vi "Synchronized Acquisition.vi"() -> ()   [LabVIEW 2021]
uses:
  <vilib>/userdefined/Silver/nirio_resource_slv.ctl
  Digitizer Control Class/Public/Acq Start Trigger Type.ctl
  <instrlib>/FlexRIO/API/Host/v1/NI FlexRIO/API/Reference Clock Source.ctl
  Digitizer Control Class/Public/TClk API Control Enable.ctl
  <instrlib>/FlexRIO/API/Host/v1/NI FlexRIO/API/Configure Reference Clock.vi
  <instrlib>/FlexRIO/API/Host/v1/NI FlexRIO API v1.lvlib
  <resource>/objmgr/sessionReference.rc
  Digitizer Control Class/Digitizer Control.lvclass
panel:
  out "Device Memory Utilization":u64[][](graph)
  out "Record index":i32
  in  "Acq # of records":i32=1
  out "actual pre-trigger period (s)":dbl format="%#_6p"
  in  "pre-trigger period (s)":dbl format="%#_6p"
  in  "Acq # of samples (per channel)":i64[](array[numeric])=[100000, 100000]
  in  "Enable Bit Packing (per channel)":bool[](array[boolean])=[FALSE, FALSE]
  in  "digital high level?":bool=TRUE
  in  "trigger type":T1
  in  "analog trigger channel":string="AI0"
  in  "analog/digital rising edge?":bool=TRUE
  in  "analog level (V)":dbl format="%#_3p"
  in  "analog hysteresis (V)":dbl format="%#_3p"
  in  "digital trigger source":string(combo)="DIO"
  out "Acq Overflow":bool[](array[boolean])
  in  "min. TClk period":dbl=1e-06 format="%#_6p"
  in  "trigger master index":i32
  out "Error Out":errorcluster
  in  "reference clock source":T2 items=["Default", "Onboard", "PXI_Clk10", "External", "None", "Baseboard Reference"]
  in  "Desired Sampling Rate (per device)":dbl[](array[numeric])=[800000000.0] format="%#_6p"
  out "Actual Sampling Rate (per device)":dbl[](array[numeric]) format="%#_6p"
  in  "AI channel":string="AI0,AI1"
  in  "devices":T3[](array[typedef])=["RIO0", "RIO1"]
  out "Power Spectrum":cluster{"f0":dbl, "df":dbl, "magnitude":dbl[]}[](graph) caption="Waveform Graph"
  in  "stop":bool
  out "Waveform Graph":waveform(dbl)[](graph)
  in  "TClk trigger\ncompensation?":bool
  # "Overview: Configure multiple 5774s for synchronized acquisition.\nRequirements: PXIe-5774 (KU060)\nInstructions: \n 1. Fill in the devices array with the resource name of the FlexRIO digitizers to synchronize.\n 2. Specify which device should be used as the trigger master using trigger master index\n 3. Configure the trigger settings for the master device\n 4. Optionally configure the reference clock to be used\n 5. Configure the channel to use, the number of samples and the sampling rate\n 5. Run the VI"
  # "Acquisition Trigger"
  # "Clocking configuration"
  # "Acquisition Configuration"
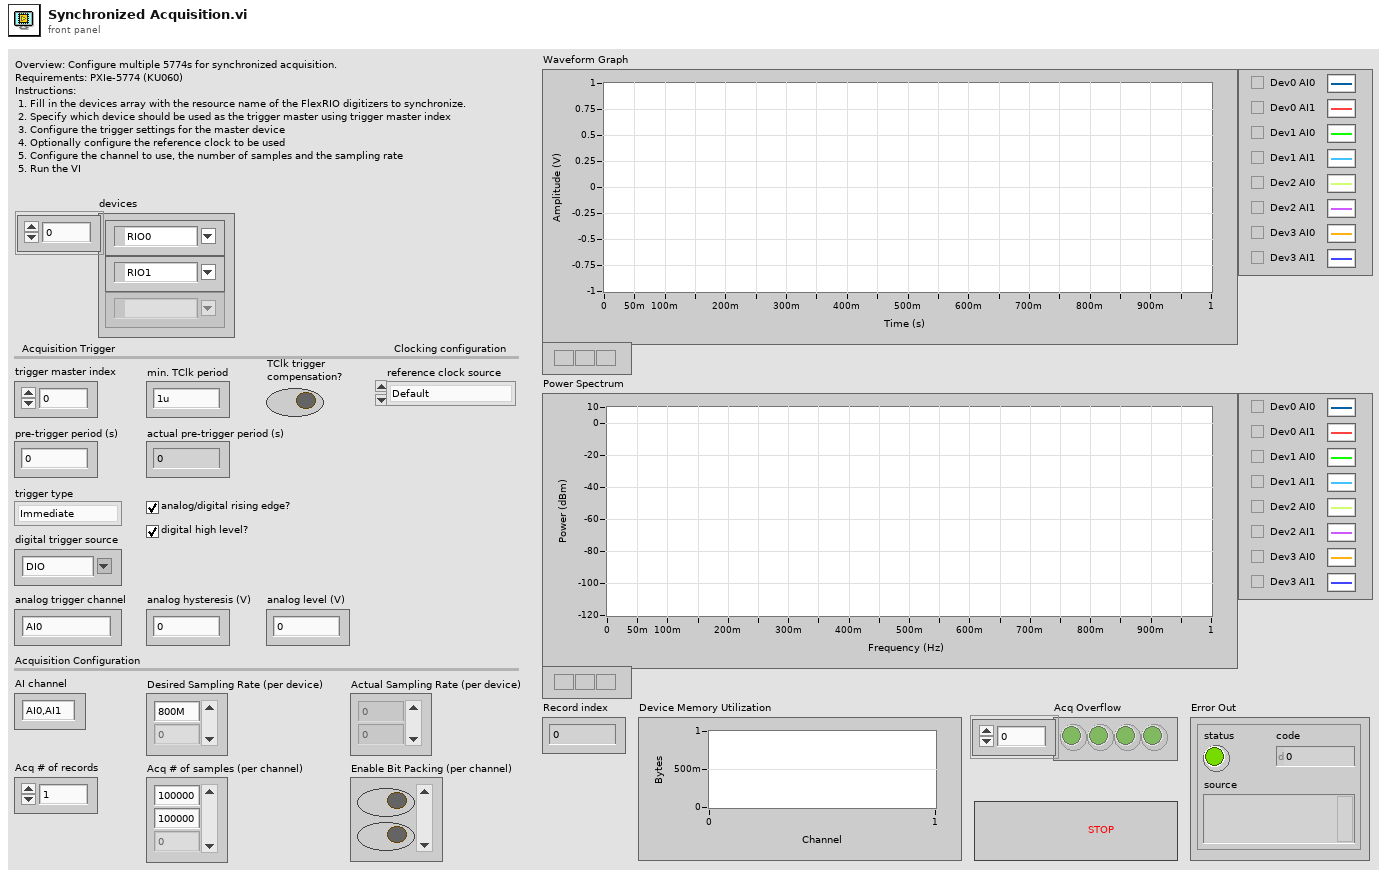
[diagram p1: front panel]
types:
  T1 = typedef "Digitizer Control.lvclass/Acq Start Trigger Type.ctl" = enum16{"Immediate", "Analog", "Digital Edge", "Digital Level"}
  T2 = typedef "NI FlexRIO API v1.lvlib/Reference Clock Source.ctl" = i32
  T3 = typedef "nirio_resource_slv.ctl" = tag
  T4 = typedef "Digitizer Control.lvclass/TClk API Control Enable.ctl" = enum16{"None", "Acquisition"}
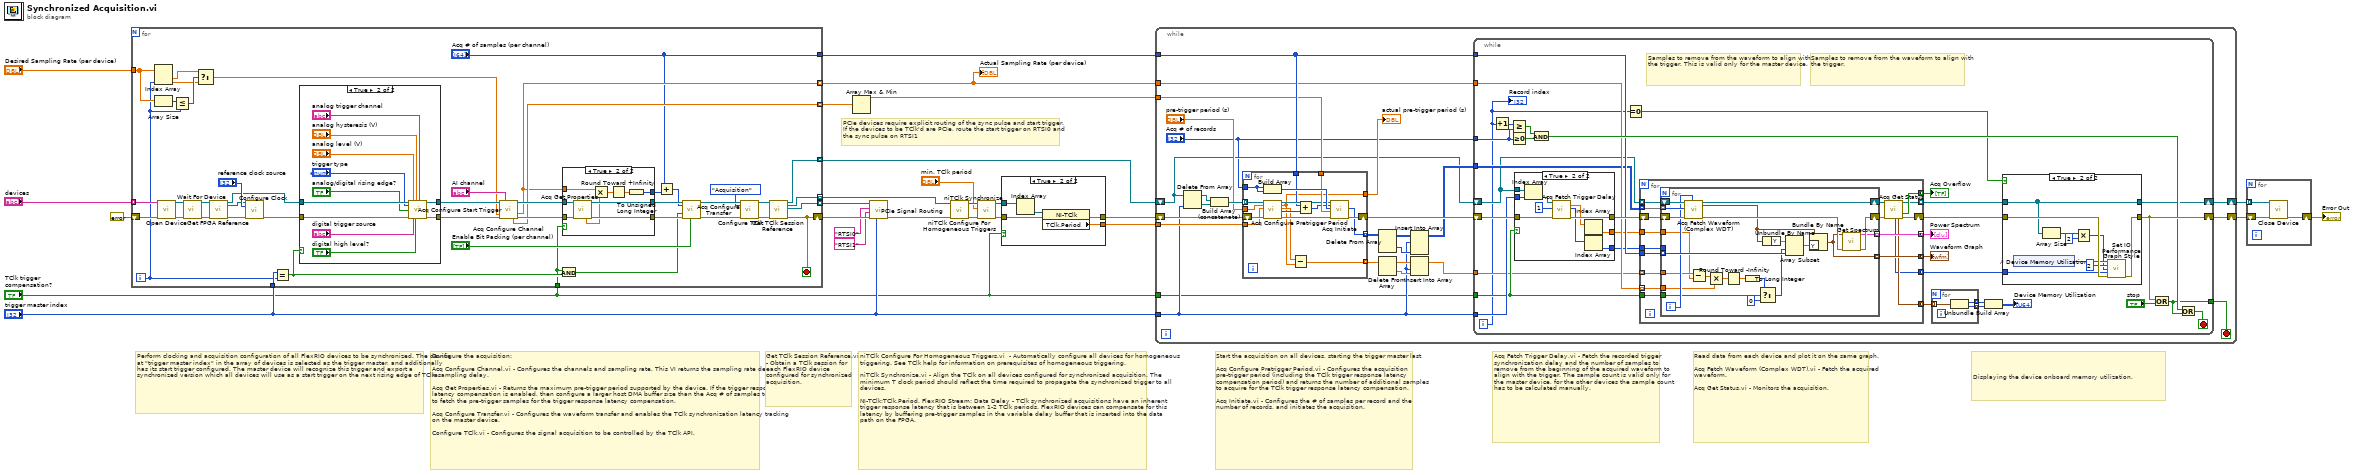
[diagram p0: block diagram]
diagram:
  # "Displaying the device onboard memory utilization."
  # "Read data from each device and plot it on the same graph.\n\nAcq Fetch Waveform (Complex WDT).vi - Fetch the acquired waveform.\n\nAcq Get Status.vi - Monitors the acquisition."
  # "Acq Fetch Trigger Delay.vi - Fetch the recorded trigger synchronization delay and the number of samples to remove from the beginning of the acquired waveform to align with the trigger. The sample count is valid only for the master device, for the other devices the sample count has to be calculated manually."
  # "Start the acquisition on all devices, starting the trigger master last\n\nAcq Configure Pretrigger Period.vi - Configures the acquisition pre-trigger period (including the TClk trigger response latency compensation period) and returns the number of additional samples to acquire for the TClk trigger response latency compensation.\n\nAcq Initiate.vi - Configures the # of samples per record and the number of records, and initiates the acquisition."
  # "Configure the acquisition:\n\nAcq Configure Channel.vi - Configures the channels and sampling rate. This VI returns the sampling rate dependent resampling delay.\n\nAcq Get Properties.vi - Returns the maximum pre-trigger period supported by the device. If the trigger response latency compensation is enabled, then configure a larger host DMA buffer size than the Acq # of samples to be able to fetch the pre-trigger samples for the trigger response latency compensation.\n\nAcq Configure Transfer.vi - Configures the waveform transfer and enables the TClk synchronization latency tracking on the master device.\n\nConfigure TClk.vi - Configures the signal acquisition to be controlled by the TClk API."
  # "PCIe devices require explicit routing of the sync pulse and start trigger.\nIf the devices to be TClk'd are PCIe, route the start trigger on RTSI0 and\nthe sync pulse on RTSI1"
  # "Get TClk Session Reference.vi  - Obtain a TClk session for each FlexRIO device configured for synchronized acquisition."
  # "Perform clocking and acquisition configuration of all FlexRIO devices to be synchronized. The device at \"trigger master index\" in the array of devices is selected as the trigger master, and additionally has its start trigger configured. The master device will recognize this trigger and export a synchronized version which all devices will use as a start trigger on the next rising edge of TClk."
  # "niTClk Configure For Homogeneous Triggers.vi  - Automatically configure all devices for homogeneous triggering. See TClk help for information on prerequisites of homogeneous triggering. \n\nniTClk Synchronize.vi - Align the TClk on all devices configured for synchronized acquisition. The minimum T clock period should reflect the time required to propagate the synchronized trigger to all devices. \n\nNI-TClk:TClk.Period, FlexRIO Stream: Data Delay - TClk synchronized acquisitions have an inherent trigger response latency that is between 1-2 TClk periods. FlexRIO devices can compensate for this latency by buffering pre-trigger samples in the variable delay buffer that is inserted into the data path on the FPGA."
  n1 = for {
    tunnel: "devices" -> [w57] mode=indexing
    tunnel: [w46] -> w17 mode=indexing
    tunnel: [w45] -> w11 mode=indexing
    shift-right: [w30] -> w26
    shift-left: errorcluster {"status"=FALSE, "code"=0, "source"=""} ("error out") -> [w58]
    tunnel: "trigger master index" -> [w60]
    tunnel: [w44] -> w4 mode=indexing
    tunnel: [w35] -> w9 mode=indexing
    tunnel: "Desired Sampling Rate (per device)" -> [w37]
    tunnel: [w38] -> w7 mode=indexing
    tunnel: ["Acq # of samples (per channel)"] -> w2
    tunnel: "TClk trigger\ncompensation?" -> [w27]
    i -> [w31]
    stop <- w30 stop-if-true
    n2 = Index Array(array=w37, index #2=w31) -> (element #1=w41:dbl, element #2=w40:dbl)  [unwired: 1 in]
    n3 = Array Size(array=w37) -> (size(s)=w43:i32)
    n4 = call "Open Device.vi"("resource name"=w57, "error in (no error)"=w58) -> ("session out"=w55:refnum<class "Digitizer Control.lvclass">, "error out"=w56:errorcluster)  [unwired: 16 in]
    n5 = Less Or Equal?(x=w43, y=w31) -> (x <= y?=w42:bool)
    n6 = call "Wait For Device.vi"("session in"=w55, "error in (no error)"=w56) -> ("session out"=w53:refnum<class "Digitizer Control.lvclass">, "error out"=w54:errorcluster)  [unwired: 15 in, 1 out]
    n7 = Select(t=w41, s=w42, f=w40) -> (s? t:f=w39:dbl)
    n8 = call "Get FPGA Reference.vi"("session in"=w53, "error in (no error)"=w54) -> ("session out"=w52:refnum<class "Digitizer Control.lvclass">, "fpga reference"=w51:refnum<k20>, "error out"=w50:errorcluster)  [unwired: 15 in]
    n9 = call-poly <instrlib>:"Configure Clock.vi"("fpga interface in"=w51, "reference clock source"="reference clock source", "error in"=w50) -> ("error out"=w49:errorcluster)  [unwired: 11 in, 1 out]
    n10 = Equal?(x=w60, y=w31) -> (x = y?=w29:bool)
    n11 = case shown="True" w29 {
      tunnel: w49 -> [w82 w94]
      tunnel: w52 -> [w83 w93]
      tunnel: [w82 w91] -> w64
      tunnel: [w83 w92] -> w48
      frame False {
      }
      frame True {
        n12 = call "Acq Configure Start Trigger.vi"("session in"=w93, "trigger type (Immediate)"="trigger type", "rising edge? (T)"="analog/digital rising edge?", "error in (no error)"=w94, "analog level (0)"="analog level (V)", "digital trigger source (PXI_Trig0)"="digital trigger source", "analog hysteresis (0)"="analog hysteresis (V)", "digital high level? (T)"="digital high level?", "analog trigger channel (AI0)"="analog trigger channel") -> ("session out"=w92:refnum<class "Digitizer Control.lvclass">, "error out"=w91:errorcluster)  [unwired: 9 in]
      }
    }
    n13 = call "Acq Configure Channel.vi"("session in"=w48, "sampling rate (SPS)"=w39, "error in (no error)"=w64, "AI channel"="AI channel") -> ("DSP delay (s)"=w38:dbl, "session out"=w70:refnum<class "Digitizer Control.lvclass">, "actual sampling rate (SPS)"=w35:dbl, "error out"=w68:errorcluster)  [unwired: 9 in, 3 out]
    n14 = And(x=w27, y=w29) -> (x .and. y?=w28:bool)
    n15 = case shown="True" w27 {
      tunnel: w68 -> [w71 w79]
      tunnel: w70 -> [w72 w81]
      tunnel: [w72 w80] -> w69
      tunnel: [w71 w78] -> w67
      tunnel: [_ w77] -> w36
      tunnel: w35 -> [_ w74]
      frame False {
      }
      frame True {
        n16 = call "Acq Get Properties.vi"("session in"=w81, "error in (no error)"=w79) -> ("maximum pre-trigger period (s)"=w73:dbl, "session out"=w80:refnum<class "Digitizer Control.lvclass">, "error out"=w78:errorcluster)  [unwired: 15 in]
        n17 = Multiply(x=w74, y=w73) -> (x*y=w75:dbl)
        n18 = Round Toward +Infinity(x=w75) -> (ceil(x): smallest int >= x=w76:dbl)
        n19 = To Unsigned Long Integer(number=w76) -> (unsigned 32bit integer=w77:u32)
      }
    }
    n20 = Add(x="Acq # of samples (per channel)", y=w36) -> (x+y=w34:i64[])
    n21 = call "Acq Configure Transfer.vi"("session in"=w69, "host DMA buffer size (samples)"=w34, "trigger delay tracking enable (F)"=w28, "error in (no error)"=w67, "enable bit packing (F)"="Enable Bit Packing (per channel)") -> ("session out"=w65:refnum<class "Digitizer Control.lvclass">, "error out"=w66:errorcluster)  [unwired: 8 in, 5 out]
    n22 = call "Configure TClk.vi"("session in"=w65, "TClk API Control Enable"=TClk_API_Control_Enable."Acquisition", "error in (no error)"=w66) -> ("session out"=w47:refnum<class "Digitizer Control.lvclass">, "error out"=w63:errorcluster)  [unwired: 15 in]
    n23 = call "Get TClk Session Reference.vi"("session in"=w47, "error in (no error)"=w63) -> ("session out"=w44:refnum<class "Digitizer Control.lvclass">, "tclk session reference"=w45:refnum<k20>, "fpga reference"=w46:refnum<k20>, "error out"=w30:errorcluster)  [unwired: 14 in]
  }
  "Actual Sampling Rate (per device)" <- w9
  n24 = Array Max & Min(array=w7) -> (max value=w6:dbl)  [unwired: 3 out]
  n25 = call "PCIe Signal Routing.vi"("trigger master index"="trigger master index", "error in (no error)"=w26, "sync pulse rtsi line"="RTSI1", "start trigger rtsi line"="RTSI0", "fpga interfaces in"=w17) -> ("error out"=w25:errorcluster)  [unwired: 5 in, 1 out]
  n26 = call <instrlib>:"niTClk Configure For Homogeneous Triggers.vi"("error in (no error)"=w25, "sessions"=w11) -> ("error out"=w24:errorcluster, "sessions out"=w23:refnum<k20>[])  [unwired: 8 in]
  n27 = call <instrlib>:"niTClk Synchronize.vi"("error in (no error)"=w24, "minimum T clock period"="min. TClk period", "sessions"=w23) -> ("error out"=w22:errorcluster, "sessions out"=w21:refnum<k20>[])  [unwired: 7 in]
  n28 = case shown="True" "TClk trigger\ncompensation?" {
    tunnel: w22 -> [w95 w100]
    tunnel: w21 -> [_ w98]
    tunnel: [w95 w96] -> w3
    tunnel: [_ w97] -> w5
    frame False {
    }
    frame True {
      n29 = Index Array(array=w98) -> (element=w99:refnum<k20>)  [unwired: 1 in]
      n30 = property class="NI-TClk"(reference=w99, error in=w100) -> (error out=w96:errorcluster, "TClk.Period"=w97:dbl)  [unwired: 1 out]
    }
  }
  n31 = while {
    shift-right: [w121] -> w19
    shift-left: w3 -> [w126]
    shift-right: [w104] -> w18
    shift-left: w4 -> [w103]
    tunnel: "trigger master index" -> [w107]
    tunnel: "TClk trigger\ncompensation?" -> [w106]
    tunnel: w9 -> [w123]
    tunnel: w6 -> [w117]
    tunnel: w5 -> [w116]
    tunnel: w2 -> [w124]
    stop <- w101 stop-if-true
    n32 = Delete From Array(array=w103, index=w107) -> (deleted portion=w119:refnum<class "Digitizer Control.lvclass">, array with subset deleted=w120:refnum<class "Digitizer Control.lvclass">[])  [unwired: 1 in]
    n33 = Build Array (concatenate)(w120, w119) -> (w118:refnum<class "Digitizer Control.lvclass">[])
    n34 = for {
      tunnel: w118 -> [w237] mode=indexing
      shift-right: [w241] -> w125
      shift-left: w126 -> [w240]
      tunnel: [w226] -> w113 mode=indexing
      tunnel: w117 -> [w238]
      tunnel: w116 -> [w236]
      tunnel: "pre-trigger period (s)" -> [w235]
      tunnel: w124 -> [w232]
      tunnel: [w229] -> w114
      tunnel: [w228] -> w112 mode=indexing
      tunnel: "Acq # of records" -> [w227]
      n35 = Build Array(w227, w227) -> (w242:i32[])
      n36 = call "Acq Configure Pretrigger Period.vi"("session in"=w237, "desired pre-trigger period (s)"=w235, "TClk period (s)"=w236, "error in (no error)"=w240) -> ("session out"=w234:refnum<class "Digitizer Control.lvclass">, "actual pre-trigger period (s)"=w229:dbl, "configured pre-trigger period (s)"=w230:dbl, "additional samples to acquire (samples)"=w233:i64, "error out"=w239:errorcluster)  [unwired: 11 in]
      n37 = Subtract(x=w230, y=w229) -> (x-y=w228:dbl)
      n38 = Add(x=w232, y=w233) -> (x+y=w231:i64[])
      n39 = call "Acq Initiate.vi"("session in"=w234, "sample count (-1)"=w231, "record count (1)"=w242, "desired delay (s)"=w238, "error in (no error)"=w239) -> ("elements to read"=w226:i64[], "error out"=w241:errorcluster)  [unwired: 8 in, 5 out]
    }
    "actual pre-trigger period (s)" <- w114
    n40 = Delete From Array(array=w113) -> (deleted portion=w110:i64[], array with subset deleted=w111:i64[][])  [unwired: 3 in]
    n41 = Delete From Array(array=w112) -> (deleted portion=w108:dbl, array with subset deleted=w109:dbl[])  [unwired: 2 in]
    n42 = Insert Into Array(array=w111, index (row)=w107, new element=w110) -> (w122:i64[][])  [unwired: 1 in]
    n43 = Insert Into Array(array=w109, index=w107, new element=w108) -> (w105:dbl[])
    n44 = while {
      tunnel: w124 -> [w154]
      tunnel: w123 -> [w153]
      tunnel: w122 -> [w152]
      tunnel: w107 -> [w146]
      tunnel: w106 -> [w144]
      tunnel: w105 -> [w143]
      shift-right: [w158] -> w121
      shift-left: w125 -> [w156]
      shift-right: [w131] -> w104
      shift-left: w103 -> [w150]
      tunnel: [w128] -> w101
      tunnel: "Acq # of records" -> [w141]
      i -> [w138]
      stop <- w127 stop-if-true
      # "Samples to remove from the waveform to align with the trigger."
      # "Samples to remove from the waveform to align with the trigger. This is valid only for the master device."
      n45 = Increment(x=w138) -> (x+1=w142:i32)
      n46 = Greater Or Equal?(x=w142, y=w141) -> (x >= y?=w140:bool)
      n47 = Greater Or Equal To 0?(x=w141) -> (x >= 0?=w139:bool)
      n48 = case shown="True" w144 {
        tunnel: w150 -> [_ w182]
        tunnel: w146 -> [_ w181]
        tunnel: w156 -> [w174 w184]
        tunnel: [w174 w183] -> w155
        tunnel: [_ w177] -> w149
        tunnel: [_ w175] -> w145
        frame False {
        }
        frame True {
          n49 = Index Array(array=w182, index=w181) -> (element=w180:refnum<class "Digitizer Control.lvclass">)
          n50 = call "Acq Fetch Trigger Delay.vi"("session in"=w180, "records to read"=u32 1, "error in (no error)"=w184) -> ("trigger delay (s)"=w176:dbl[], "samples to ignore"=w178:i32[], "error out"=w183:errorcluster)  [unwired: 12 in, 2 out]
          n51 = Index Array(array=w176) -> (element=w175:dbl)  [unwired: 1 in]
          n52 = Index Array(array=w178) -> (element=w177:i32)  [unwired: 1 in]
        }
      }
      n53 = And(x=w140, y=w139) -> (x .and. y?=w157:bool)
      n54 = Equal To 0?(x=w138) -> (x = 0?=w130:bool)
      n55 = for {
        tunnel: w150 -> [w201] mode=indexing
        shift-right: [w196] -> w159
        shift-left: w155 -> [w202]
        tunnel: w152 -> [w185] mode=indexing
        tunnel: [w200] -> w151 mode=concatenating
        tunnel: [w199] -> w133 mode=indexing
        tunnel: [w195] -> w147 mode=concatenating
        tunnel: w149 -> [w194]
        tunnel: w154 -> [w193]
        tunnel: [w192] -> w148 mode=concatenating
        tunnel: w145 -> [w191]
        tunnel: w144 -> [w190]
        tunnel: w143 -> [w189] mode=indexing
        tunnel: w153 -> [w188] mode=indexing
        tunnel: [w187] -> w137 mode=concatenating
        tunnel: [w186] -> w132 mode=concatenating
        n56 = for {
          tunnel: w185 -> [w221] mode=indexing
          shift-right: [w220] -> w198
          shift-left: w201 -> [w222]
          shift-right: [w223] -> w197
          shift-left: w202 -> [w224]
          tunnel: [w215] -> w195 mode=indexing
          tunnel: w194 -> [_]
          tunnel: w193 -> [w216] mode=indexing
          tunnel: [w214] -> w192 mode=indexing
          tunnel: w191 -> [w211]
          tunnel: w190 -> [w206]
          tunnel: w189 -> [w212]
          tunnel: w188 -> [w209]
          i -> [w213]
          n57 = call "Acq Fetch Waveform (Complex WDT).vi"("session in"=w222, "elements to read"=w221, "error in (no error)"=w224, "channel index"=w213) -> ("session out"=w220:refnum<class "Digitizer Control.lvclass">, "waveform (V)"=w217:waveform(dbl), "error out"=w225:errorcluster)  [unwired: 11 in, 2 out]
          n58 = Subtract(x=w212, y=w211) -> (x-y=w210:dbl)
          n59 = Multiply(x=w210, y=w209) -> (x*y=w208:dbl)
          n60 = Round Toward -Infinity(1:w208) -> (0:w207:dbl)
          n61 = To Long Integer(number=w207) -> (32bit integer=w205:i32)
          n62 = Select(t=w205, s=w206, f=0) -> (s? t:f=w203:i32)
          n63 = Unbundle By Name(w217) -> ("Y"=w218:dbl[])
          n64 = Array Subset(array=w218, index=w203, length=w216) -> (w219:dbl[])
          n65 = Bundle By Name(cluster=w217, "Y"=w219) -> (w215:waveform(dbl))
          n66 = call "Get Spectrum.vi"("waveform (V)"=w215, "error in (no error)"=w225) -> ("power spectrum (dBm)"=w214:cluster{"f0":dbl, "df":dbl, "magnitude":dbl[]}, "error out"=w223:errorcluster)  [unwired: 12 in]
        }
        n67 = call "Acq Get Status.vi"("session in"=w198, "error in (no error)"=w197) -> ("memory size"=w186:u64[], "memory utilization"=w187:cluster{"lowest":u64, "highest":u64}[], "session out"=w199:refnum<class "Digitizer Control.lvclass">, "overflow"=w200:bool[], "error out"=w196:errorcluster)  [unwired: 8 in, 5 out]
      }
      "Acq Overflow" <- w151
      "Waveform Graph" <- w147
      "Power Spectrum" <- w148
      n68 = for {
        tunnel: w137 -> [w173] mode=indexing
        tunnel: [w172] -> w136 mode=indexing
        tunnel: [w171] -> w135 mode=indexing
        n69 = Unbundle(w173) -> ("lowest"=w172:u64, "highest"=w171:u64)
      }
      n70 = Build Array(w136, w135) -> (→"Device Memory Utilization":u64[][])
      n71 = case shown="True" w130 {
        tunnel: w159 -> [w160 w170]
        tunnel: [w160 w169] -> w158
        tunnel: w133 -> [w161 w164]
        tunnel: w132 -> [_ w165]
        tunnel: [w161 w164] -> w131
        frame False {
        }
        frame True {
          n72 = control-ref of="Device Memory Utilization"() -> (w168:refnum<vi>)
          n73 = Array Size(array=w164) -> (size(s)=w166:i32)
          n74 = Multiply(x=w166, y=2) -> (x*y=w163:i32)
          n75 = call "Set IO Performance Graph Style.vi"("Waveform Graph Refnum"=w168, "# of plots (1)"=2, "# of devices (1)"=w163, "Y maximum (1)"=w165, "error in (no error)"=w170) -> ("error out"=w169:errorcluster)  [unwired: 10 in]
        }
      }
      n76 = Or(x=w158, y="stop") -> (x .or. y?=w128:bool)
      n77 = Or(x=w157, y=w128) -> (x .or. y?=w127:bool)
      "Record index" <- w138
    }
  }
  n78 = for {
    tunnel: w18 -> [w244] mode=indexing
    shift-right: [w243] -> w13
    shift-left: w19 -> [w245]
    n79 = call "Close Device.vi"("session in"=w244, "error in (no error)"=w245) -> ("error out"=w243:errorcluster)  [unwired: 17 in]
  }
  "Error Out" <- w13
